vi "COMMAND_ChangeVelocity.vi"(8 "error in (no error)":errorcluster, 10 "configuration data.speed":dbl[unit][](array[numeric]), 11 "MH100301DMC in":refnum<class "StageMH100301DMC.lvclass">) -> (0 "error out":errorcluster, 3 "MH100301DMC out":refnum<class "StageMH100301DMC.lvclass">)   [LabVIEW 2010, in "StageMH100301DMC.lvclass"]
uses:
  StageMH100301DMC.lvclass
  StageMH100301DMC.lvclass/StageMH100301DMC.ctl
  common/classes/ErrorController/ErrorController/class_data.vi
  common/classes/ErrorController/ErrorController/ErrorController.lvclass
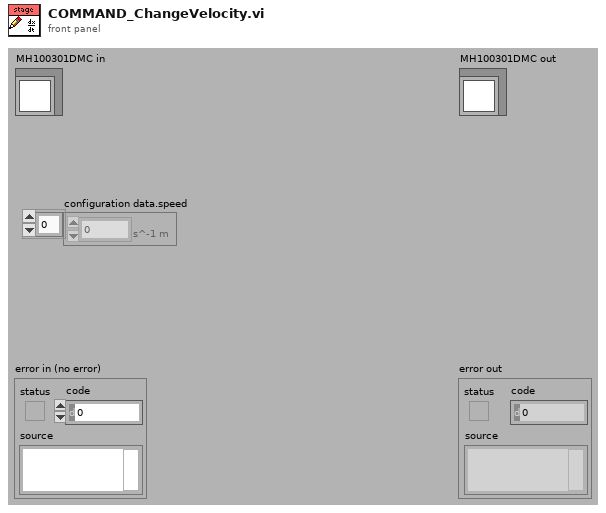
[diagram p1: front panel]
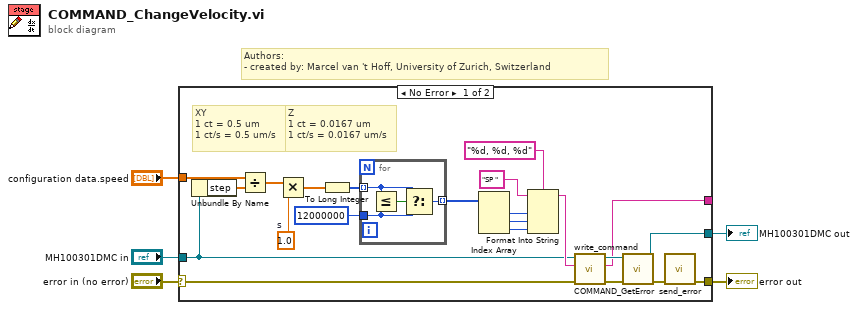
[diagram p0: block diagram]
diagram:
  # "Authors: \n- created by: Marcel van 't Hoff, University of Zurich, Switzerland"
  n1 = case shown="No Error" "error in (no error)" {
    selector: "error in (no error)" -> [w27 w33]
    tunnel: [w6 w33] -> w4
    tunnel: [w12 w32] -> w2
    tunnel: "MH100301DMC in" -> [w17 w32]
    tunnel: "configuration data.speed" -> [w25 _]
    tunnel: [w9 _] -> _
    frame No Error {
      w8 = dbl[unit] 1.0  # s
      # "XY\n1 ct = 0.5 um\n1 ct/s = 0.5 um/s"
      # "Z\n1 ct = 0.0167 um\n1 ct/s = 0.0167 um/s"
      n2 = Unbundle By Name(w17) -> ("step"=w26:dbl[unit][])
      n3 = Divide(x=w25, y=w26) -> (x/y=w24:dbl[unit][])
      n4 = Multiply(x=w24, y=w8) -> (x*y=w23:dbl[])
      n5 = To Long Integer(number=w23) -> (32bit integer=w19:i32[])
      n6 = for {
        tunnel: w19 -> [w31] mode=indexing
        tunnel: 12000000 ("y") -> [w30]
        tunnel: [w28] -> w10 mode=indexing
        n7 = Less Or Equal?(x=w31, y=w30) -> (x <= y?=w29:bool)
        n8 = Select(t=w31, s=w29, f=w30) -> (s? t:f=w28:i32)
      }
      n9 = Index Array(array=w10) -> (element #1=w16:i32, element #2=w15:i32, element #3=w14:i32)  [unwired: 3 in]
      n10 = Format Into String(format string="%d, %d, %d", initial string="SP ", w16, w15, w14) -> (resulting string=w20:string)  [unwired: 1 in, 1 out]
      n11 = call-dynamic "write_command.vi"("error in (no error)"=w27, "command (without terminating \"\\n\")"=w20, "MH100301DMC in"=w17) -> ("error out"=w11:errorcluster, "response out"=w9:string, "MH100301DMC out"=w13:refnum<class "StageMH100301DMC.lvclass">)  [unwired: 6 in]
      n12 = call-dynamic "COMMAND_GetError.vi"("error in (no error)"=w11, "StageMH100301DMC in"=w13) -> ("error out"=w7:errorcluster, "StageMH100301DMC out"=w12:refnum<class "StageMH100301DMC.lvclass">)  [unwired: 8 in]
      n13 = call "send_error.vi"("error in (no error)"=w7) -> ("error out"=w6:errorcluster)  [unwired: 10 in]
    }
    frame Error {
    }
  }
  "error out" <- w4
  "MH100301DMC out" <- w2
